vi "Close.vi"(8 "error in (no error)":errorcluster, 11 "MelsecTCP in":refnum<class "MelsecFxLinks.lvclass">) -> (0 "error out":errorcluster, 3 "MelsecTCP out":refnum<class "MelsecFxLinks.lvclass">)   [LabVIEW 2020, in "MelsecFxLinks.lvclass"]
uses:
  MelsecFxLinks.lvclass
  C:/Users/Fred Guo/Desktop/API_Salcomp_CMES/Libraries/HslCommunication/HslCommunication.dll
  HslCommunication.dll
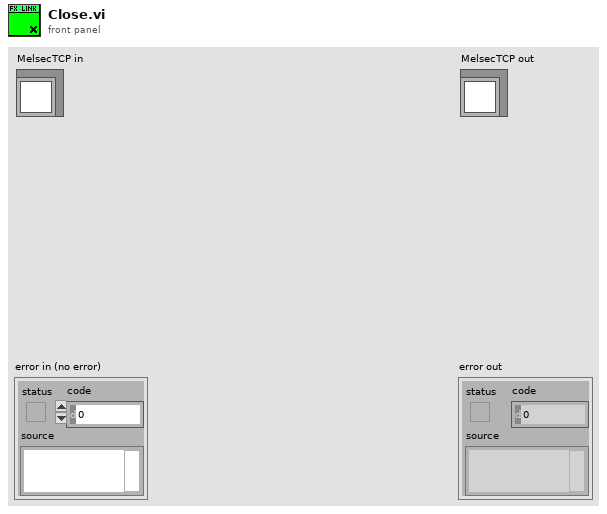
[diagram p1: front panel]
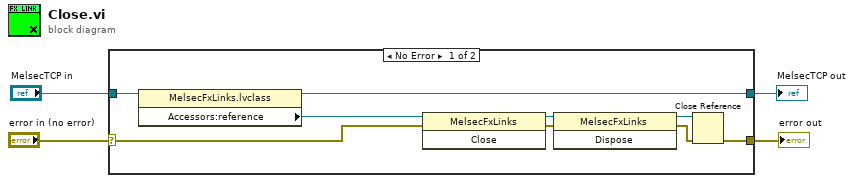
[diagram p0: block diagram]
diagram:
  n1 = case shown="No Error" "error in (no error)" {
    selector: "error in (no error)" -> [w5 w15]
    tunnel: "MelsecTCP in" -> [w13 w14]
    tunnel: [w12 w14] -> w2
    tunnel: [w11 w15] -> w1
    frame No Error {
      n2 = property class="MelsecFxLinks.lvclass"(reference=w13) -> (reference out=w12:refnum<class "MelsecFxLinks.lvclass">, "Accessors:reference"=w6:refnum<k24>)  [unwired: 1 in, 1 out]
      n3 = invoke class="MelsecFxLinks" method="Close"(reference=w6, error in=w5) -> (reference out=w8:refnum<k24>, error out=w7:errorcluster)  [unwired: 1 in, 1 out]
      n4 = invoke class="MelsecFxLinks" method="Dispose"(reference=w8, error in=w7) -> (reference out=w10:refnum<k24>, error out=w9:errorcluster)  [unwired: 1 in, 1 out]
      n5 = Close Reference(reference=w10, error in (no error)=w9) -> (error out=w11:errorcluster)
    }
    frame Error {
    }
  }
  "error out" <- w1
  "MelsecTCP out" <- w2
